vi "XML Write Scheds.vi"(8 "error in":errorcluster, 10 "File Save As":string, 11 "Sched Values":string[](array[string])) -> (0 "error out":errorcluster)   [LabVIEW 2023]
uses:
  TAGS.ctl
panel:
  out "string array":string[](array[string])
  out "File Saved":bool
  out "output cluster":cluster{"TAGLIST":T1[]}
  out "Array":cluster{"TAG":T1}[][](array[cluster])
  in  "TAG":T1[](array[typedef])
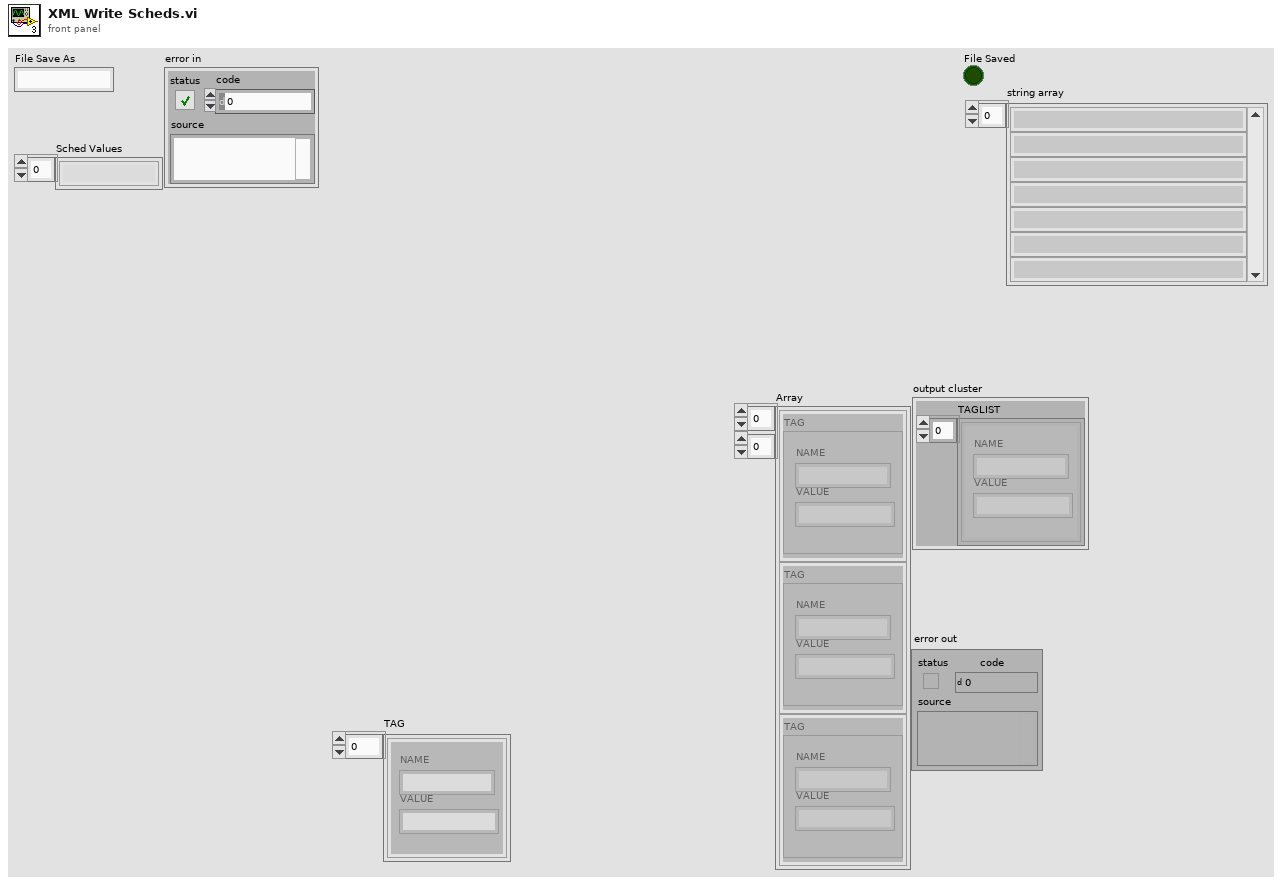
[diagram p1: front panel]
types:
  T1 = typedef "TAGS.ctl" = cluster{"NAME":string, "VALUE":string}
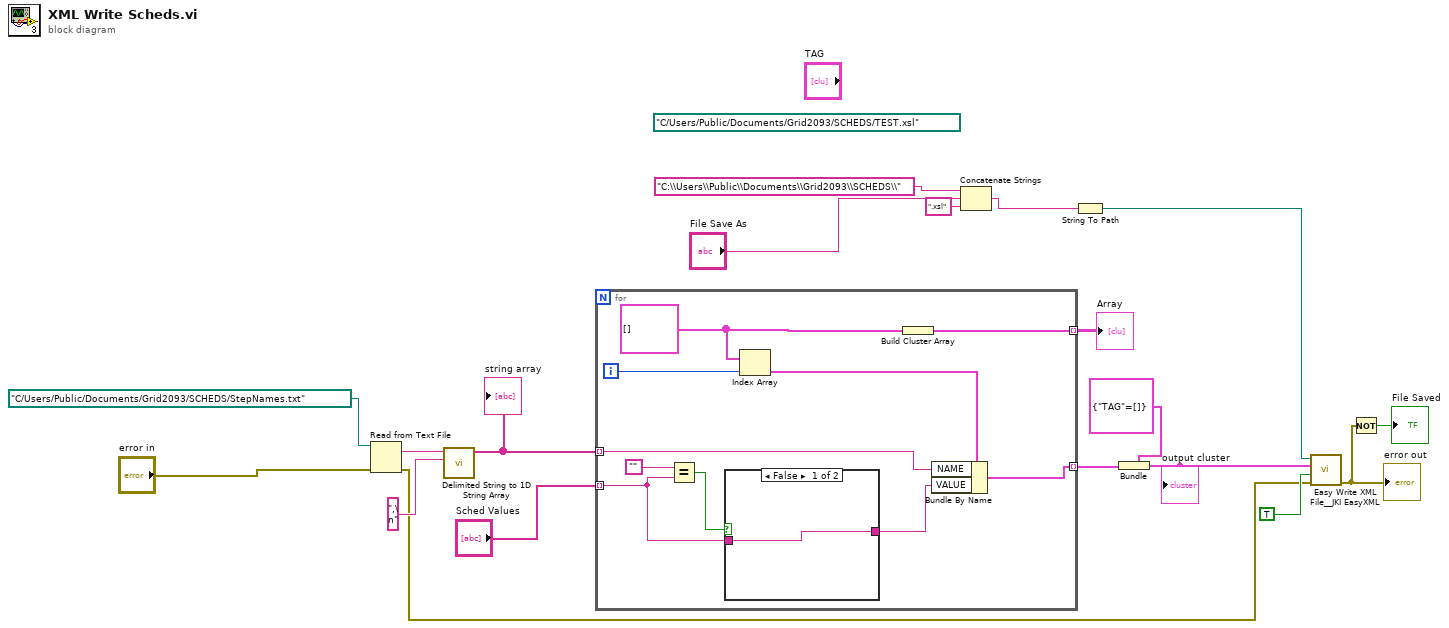
[diagram p0: block diagram]
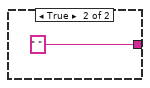
[diagram p2: hidden frame]
diagram:
  (unwired) path "C:/Users/Public/Documents/Grid2093/SCHEDS/TEST.xsl" ("XML File Path")
  n1 = Read from Text File(file (use dialog)=path "C:/Users/Public/Documents/Grid2093/SCHEDS/StepNames.txt" ("XML File Path"), error in="error in") -> (text=w5:string, error out=w1:errorcluster)  [unwired: 2 in, 2 out]
  n2 = call <vilib>:"Delimited String to 1D String Array.vi"("delimiter"=",\n", "delimited string"=w5) -> ("string array"=w3:string[])  [unwired: 9 in]
  "string array" <- w3
  n3 = for {
    tunnel: "Sched Values" -> [w20] mode=indexing
    tunnel: w3 -> [w25] mode=indexing
    tunnel: [w24] -> w16 mode=indexing
    tunnel: [w29] -> w18 mode=indexing
    i -> [w27]
    w28 = T1[] [] ("TAG")
    n4 = Equal?(x="", y=w20) -> (x = y?=w22:bool)
    n5 = case shown="False" w22 {
      tunnel: [w30 " "] -> w21
      tunnel: w20 -> [w30 _]
      frame False {
      }
      frame True {
      }
    }
    n6 = Index Array(array=w28, index=w27) -> (element=w26:T1)
    n7 = Build Cluster Array(w28) -> (w29:cluster{"TAG":T1}[])
    n8 = Bundle By Name(cluster=w26, "NAME"=w25, "VALUE"=w21) -> (w24:T1)
  }
  "Array" <- w18
  n9 = Concatenate Strings("C:\\Users\\Public\\Documents\\Grid2093\\SCHEDS\\", "File Save As", ".xsl" ("string")) -> (w9:string)
  n10 = String To Path(string=w9) -> (path=w7:path)
  n11 = Bundle(cluster=cluster{"TAG":T1[]} {"TAG"=[]} ("TAGLIST"), "TAG"=w16) -> (w17:cluster{"TAG":T1[]})
  "output cluster" <- w17
  n12 = call <vilib>:"Easy Write XML File__JKI EasyXML.vi"("error in (no error)"=w1, "Overwrite File? (false)"=TRUE, "LabVIEW Data"=w17, "XML File Path"=w7) -> ("error out"=w12:errorcluster)  [unwired: 6 in, 1 out]
  "error out" <- w12
  n13 = Not(x=w12) -> (.not. x?=→"File Saved":bool)
